vi "Set Channel Class.vi"(8 "error in":errorcluster, 11 "analog input mode in":refnum<class "Analog Input Mode.lvclass">) -> (0 "error out":errorcluster, 3 "analog input mode out":refnum<class "Analog Input Mode.lvclass">)   [LabVIEW 2017, in "Scan Engine Scripting.lvlib" / "Analog Input Mode.lvclass"]
uses:
  Analog Input Mode.lvclass
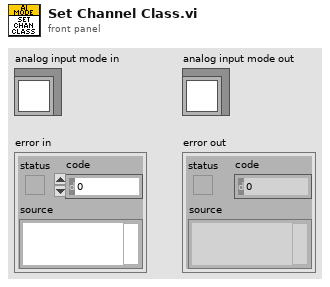
[diagram p1: front panel]
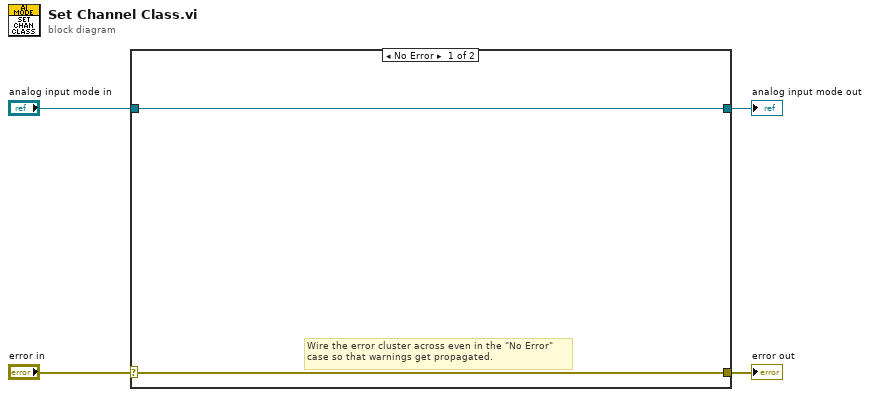
[diagram p0: block diagram]
diagram:
  n1 = case shown="No Error" "error in" {
    selector: "error in" -> [w5 w8]
    tunnel: [w5 w8] -> w3
    tunnel: [w6 w7] -> w1
    tunnel: "analog input mode in" -> [w6 w7]
    frame No Error {
      # "Wire the error cluster across even in the \"No Error\"\ncase so that warnings get propagated."
    }
    frame Error {
    }
  }
  "error out" <- w3
  "analog input mode out" <- w1
